vi "E5071C校准.vi"(4 "起始频率":dbl=947500000.0 format="%^.2e", 6 "测量点数":i32=401, 7 "终止频率":dbl=200000000.0 format="%^.2e", 9 "中频带宽":dbl=10000.0 format="%^.2e", 10 "Save State (F: Disable)":bool, 11 "VISA Refnum in":refnum<visa-resource-name>) -> ()   [LabVIEW 2011]
uses:
  Agilent ENA Series/Agilent ENA Series.lvlib
panel:
  # "kHz"
  # "MHz"
  # "MHz"
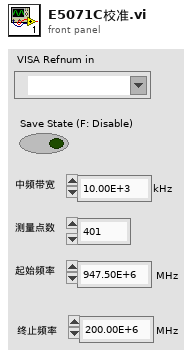
[diagram p1: front panel]
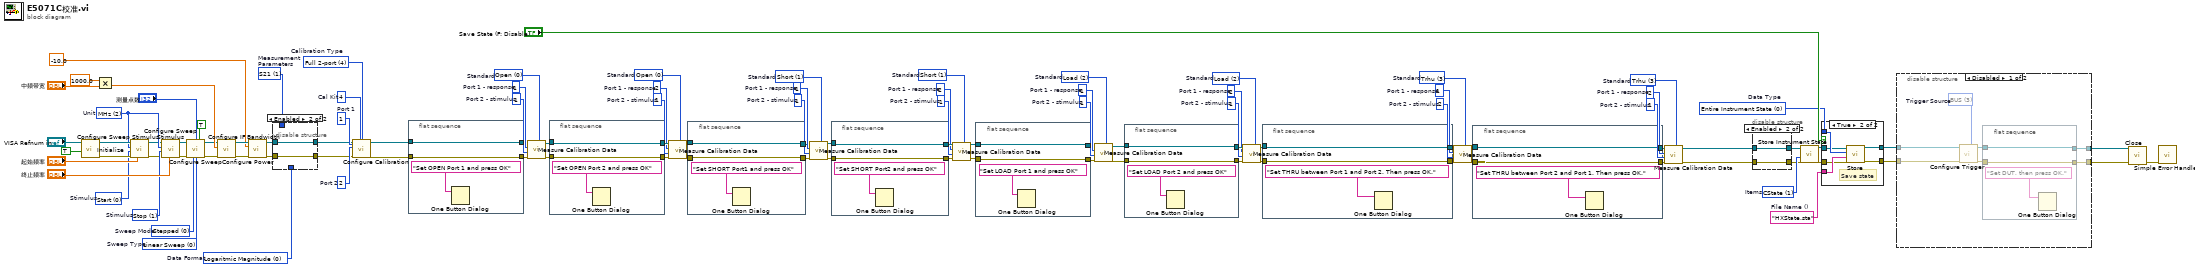
[diagram p0: block diagram]
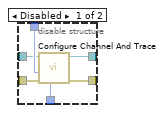
[diagram p2: hidden frame]
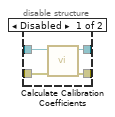
[diagram p4: hidden frame]
diagram:
  w89 = "HXState.sta"  # File Name ()
  w88 = u16 0 items=["Entire Instrument State", "Formatted Data Array", "Image On The LCD Display", "Segment Sweep Table", "Limit Table", "Power Sensor A", "Power Sensor B", "VBA Project", "Loss Compensation Table 1", "Loss Compensation Table 2", "Loss Compensation Table 3", "Loss Compensation Table 4"]  # Data Type
  w102 = u16 1 items=["State", "CState", "Dstate", "CDState"]  # Items
  w81 = u16 3 items=["Open", "Short", "Load", "Trhu", "Isolation"]  # Standard
  w79 = 1  # Port 2 - stimulus
  w80 = 2  # Port 1 - response
  w72 = u16 3 items=["Open", "Short", "Load", "Trhu", "Isolation"]  # Standard
  w76 = 2  # Port 2 - stimulus
  w75 = 1  # Port 1 - response
  w69 = u16 2 items=["Open", "Short", "Load", "Trhu", "Isolation"]  # Standard
  w65 = 1  # Port 2 - stimulus
  w66 = 2  # Port 1 - response
  w58 = u16 2 items=["Open", "Short", "Load", "Trhu", "Isolation"]  # Standard
  w62 = 1  # Port 2 - stimulus
  w61 = 1  # Port 1 - response
  w55 = u16 1 items=["Open", "Short", "Load", "Trhu", "Isolation"]  # Standard
  w51 = 1  # Port 2 - stimulus
  w52 = 2  # Port 1 - response
  w44 = u16 1 items=["Open", "Short", "Load", "Trhu", "Isolation"]  # Standard
  w48 = 1  # Port 2 - stimulus
  w47 = 1  # Port 1 - response
  w43 = u16 0 items=["Open", "Short", "Load", "Trhu", "Isolation"]  # Standard
  w42 = u16 0 items=["Open", "Short", "Load", "Trhu", "Isolation"]  # Standard
  w36 = 1  # Port 2 - stimulus
  w37 = 2  # Port 1 - response
  w35 = 1  # Port 2 - stimulus
  w34 = 1  # Port 1 - response
  w29 = 2  # Port 2
  w28 = 1  # Port 1
  w27 = u16 4 items=["Open", "Short", "Through", "1-port", "Full 2-port", "Full 3-port", "Full 4-port"]  # Calibration Type
  w26 = 4  # Cal Kit
  w23 = u16 0 items=["Logaritmic Magnitude", "Phase", "Group Delay", "Smith Chart  Linear (Lin/Phase)", "Smith Chart  Logaritmic (Log/Phase)", "Smith Chart  Complex (Real/Imag)", "Smith Chart  Impedance (R+jX)", "Smith Chart  Admittance (G+jB)", "Polar Format (Linear)", "Polar Format (Logaritmic)", "Polar Format (Re/Im)", "Linear Magnitude", "SWR", "Real", "Imaginary", "Epanded Phase", "Positive Phase"]  # Data Format
  w22 = u16 1 items=["S11", "S21", "S31", "S41", "S12", "S22", "S32", "S42", "S13", "S23", "S33", "S43", "S14", "S24", "S34", "S44", "A", "B", "C", "D", "R1", "R2", "R3", "R4"]  # Measurement Parameters
  w11 = u16 0 items=["Linear Sweep", "Logaritmic Sweep", "Segment Sweep", "Power Sweep"]  # Sweep Type
  w9 = u16 0 items=["Stepped", "Swept", "Fast Stepped Mode", "Fast Swept Mode"]  # Sweep Mode
  w6 = u16 1 items=["Start", "Stop", "Center", "Span"]  # Stimulus
  w8 = u16 2 items=["Hz", "kHz", "MHz", "GHz", "dBm", "s"]  # Unit
  w2 = u16 0 items=["Start", "Stop", "Center", "Span"]  # Stimulus
  n1 = call "Initialize.vi"("Reset? (T: Yes)"=TRUE, "VISA resource name"="VISA Refnum in") -> ("error out"=w87:errorcluster, "VISA resource name out"=w86:refnum<visa-resource-name>)  [unwired: 8 in]
  n2 = Multiply(x=1000.0, y="中频带宽") -> (x*y=w105:dbl)
  n3 = call "Configure Sweep Stimulus.vi"("Parameter (0.0)"="起始频率", "error in (no error)"=w87, "Stimulus (0: Start)"=w2, "Unit (0: Hz)"=w8, "VISA resource name"=w86) -> ("error out"=w4:errorcluster, "VISA resource name out"=w5:refnum<visa-resource-name>)  [unwired: 5 in]
  n4 = call "Configure Sweep Stimulus.vi"("Parameter (0.0)"="终止频率", "error in (no error)"=w4, "Stimulus (0: Start)"=w6, "Unit (0: Hz)"=w8, "VISA resource name"=w5) -> ("error out"=w12:errorcluster, "VISA resource name out"=w13:refnum<visa-resource-name>)  [unwired: 5 in]
  n5 = call "Configure Sweep.vi"("VISA resource name"=w13, "Number of Measurement Points (201)"="测量点数", "Auto Sweep Time (F: Off)"=TRUE, "error in (no error)"=w12, "Sweep Mode (0: Stepped)"=w9, "Sweep Type (0: Linear Sweep)"=w11) -> ("VISA resource name out"=w15:refnum<visa-resource-name>, "error out"=w16:errorcluster)  [unwired: 8 in]
  n6 = call "Configure IF Bandwidth.vi"("error in (no error)"=w16, "IF Bandwidth (100000.0)"=w105, "VISA resource name"=w15) -> ("error out"=w18:errorcluster, "VISA resource name out"=w19:refnum<visa-resource-name>)  [unwired: 7 in]
  n7 = call "Configure Power.vi"("VISA resource name"=w19, "Power Level (0.0)"=-10.0 ("Power (dBm)"), "error in (no error)"=w18) -> ("VISA resource name out"=w20:refnum<visa-resource-name>, "error out"=w21:errorcluster)  [unwired: 11 in]
  n8 = disable-structure shown="Enabled" {
    disable-tunnel: [w112 w113] -> w25
    disable-tunnel: [w111 w114] -> w24
    disable-tunnel: w23 -> [w110 _]
    disable-tunnel: w22 -> [w109 _]
    disable-tunnel: w21 -> [w108 w113]
    disable-tunnel: w20 -> [w107 w114]
    frame Disabled {
      n9 = call "Configure Channel And Trace.vi"("Data Format (0: Logarithmic Magnitude)"=w110, "error in (no error)"=w108, "Measurement Parameters (0: S11)"=w109, "VISA resource name"=w107) -> ("error out"=w112:errorcluster, "VISA resource name out"=w111:refnum<visa-resource-name>)  [unwired: 6 in]
    }
    frame Enabled {
    }
  }
  n10 = call "Configure Calibration.vi"("VISA resource name"=w24, "Port 1 (1)"=w28, "Port 2 (1)"=w29, "error in (no error)"=w25, "Cal Kit (1)"=w26, "Calibration Type (6: Full 4-port)"=w27) -> ("VISA resource name out"=w30:refnum<visa-resource-name>, "error out"=w31:errorcluster)  [unwired: 12 in]
  n11 = flat-sequence {
    tunnel: w30 -> [w116]
    tunnel: w31 -> [w115]
    tunnel: [w115] -> w33
    tunnel: [w116] -> w32
    frame #0 {
      n12 = One Button Dialog(message="Set OPEN Port 1 and press OK") -> ()  [unwired: 1 in, 1 out]
    }
  }
  n13 = call "Measure Calibration Data.vi"("Standard (0: Open)"=w42, "error in (no error)"=w33, "Port 2 - stimulus (2)"=w35, "Port 1 - response (1)"=w34, "VISA resource name"=w32) -> ("error out"=w41:errorcluster, "VISA resource name out"=w40:refnum<visa-resource-name>)  [unwired: 5 in]
  n14 = flat-sequence {
    tunnel: w40 -> [w119]
    tunnel: w41 -> [w118]
    tunnel: [w118] -> w38
    tunnel: [w119] -> w39
    frame #0 {
      n15 = One Button Dialog(message="Set OPEN Port 2 and press OK") -> ()  [unwired: 1 in, 1 out]
    }
  }
  n16 = call "Measure Calibration Data.vi"("Standard (0: Open)"=w43, "error in (no error)"=w38, "Port 2 - stimulus (2)"=w36, "Port 1 - response (1)"=w37, "VISA resource name"=w39) -> ("error out"=w50:errorcluster, "VISA resource name out"=w49:refnum<visa-resource-name>)  [unwired: 5 in]
  n17 = flat-sequence {
    tunnel: w49 -> [w122]
    tunnel: w50 -> [w121]
    tunnel: [w121] -> w46
    tunnel: [w122] -> w45
    frame #0 {
      n18 = One Button Dialog(message="Set SHORT Port1 and press OK") -> ()  [unwired: 1 in, 1 out]
    }
  }
  n19 = call "Measure Calibration Data.vi"("Standard (0: Open)"=w44, "error in (no error)"=w46, "Port 2 - stimulus (2)"=w48, "Port 1 - response (1)"=w47, "VISA resource name"=w45) -> ("error out"=w57:errorcluster, "VISA resource name out"=w56:refnum<visa-resource-name>)  [unwired: 5 in]
  n20 = flat-sequence {
    tunnel: w56 -> [w125]
    tunnel: w57 -> [w124]
    tunnel: [w124] -> w53
    tunnel: [w125] -> w54
    frame #0 {
      n21 = One Button Dialog(message="Set SHORT Port2 and press OK") -> ()  [unwired: 1 in, 1 out]
    }
  }
  n22 = call "Measure Calibration Data.vi"("Standard (0: Open)"=w55, "error in (no error)"=w53, "Port 2 - stimulus (2)"=w51, "Port 1 - response (1)"=w52, "VISA resource name"=w54) -> ("error out"=w64:errorcluster, "VISA resource name out"=w63:refnum<visa-resource-name>)  [unwired: 5 in]
  n23 = flat-sequence {
    tunnel: w63 -> [w128]
    tunnel: w64 -> [w127]
    tunnel: [w127] -> w60
    tunnel: [w128] -> w59
    frame #0 {
      n24 = One Button Dialog(message="Set LOAD Port 1 and press OK") -> ()  [unwired: 1 in, 1 out]
    }
  }
  n25 = call "Measure Calibration Data.vi"("Standard (0: Open)"=w58, "error in (no error)"=w60, "Port 2 - stimulus (2)"=w62, "Port 1 - response (1)"=w61, "VISA resource name"=w59) -> ("error out"=w71:errorcluster, "VISA resource name out"=w70:refnum<visa-resource-name>)  [unwired: 5 in]
  n26 = flat-sequence {
    tunnel: w70 -> [w131]
    tunnel: w71 -> [w130]
    tunnel: [w130] -> w67
    tunnel: [w131] -> w68
    frame #0 {
      n27 = One Button Dialog(message="Set LOAD Port 2 and press OK") -> ()  [unwired: 1 in, 1 out]
    }
  }
  n28 = call "Measure Calibration Data.vi"("Standard (0: Open)"=w69, "error in (no error)"=w67, "Port 2 - stimulus (2)"=w65, "Port 1 - response (1)"=w66, "VISA resource name"=w68) -> ("error out"=w78:errorcluster, "VISA resource name out"=w77:refnum<visa-resource-name>)  [unwired: 5 in]
  n29 = flat-sequence {
    tunnel: w77 -> [w134]
    tunnel: w78 -> [w133]
    tunnel: [w133] -> w74
    tunnel: [w134] -> w73
    frame #0 {
      n30 = One Button Dialog(message="Set THRU between Port 1 and Port 2. Then press OK.") -> ()  [unwired: 1 in, 1 out]
    }
  }
  n31 = call "Measure Calibration Data.vi"("Standard (0: Open)"=w72, "error in (no error)"=w74, "Port 2 - stimulus (2)"=w76, "Port 1 - response (1)"=w75, "VISA resource name"=w73) -> ("error out"=w83:errorcluster, "VISA resource name out"=w82:refnum<visa-resource-name>)  [unwired: 5 in]
  n32 = flat-sequence {
    tunnel: w82 -> [w137]
    tunnel: w83 -> [w136]
    tunnel: [w136] -> w94
    tunnel: [w137] -> w93
    frame #0 {
      n33 = One Button Dialog(message="Set THRU between Port 2 and Port 1. Then press OK.") -> ()  [unwired: 1 in, 1 out]
    }
  }
  n34 = call "Measure Calibration Data.vi"("Standard (0: Open)"=w81, "error in (no error)"=w94, "Port 2 - stimulus (2)"=w79, "Port 1 - response (1)"=w80, "VISA resource name"=w93) -> ("error out"=w97:errorcluster, "VISA resource name out"=w96:refnum<visa-resource-name>)  [unwired: 5 in]
  n35 = disable-structure shown="Enabled" {
    disable-tunnel: w96 -> [w142 w144]
    disable-tunnel: w97 -> [w141 w143]
    disable-tunnel: [w140 w143] -> w98
    disable-tunnel: [w139 w144] -> w99
    frame Disabled {
      n36 = call "Calculate Calibration Coefficients.vi"("error in (no error)"=w141, "VISA resource name"=w142) -> ("error out"=w140:errorcluster, "VISA resource name out"=w139:refnum<visa-resource-name>)  [unwired: 8 in]
    }
    frame Enabled {
    }
  }
  n37 = call "Store Instrument State.vi"("error in (no error)"=w98, "Items (1: CState)"=w102, "VISA resource name"=w99) -> ("error out"=w101:errorcluster, "VISA resource name out"=w100:refnum<visa-resource-name>)  [unwired: 7 in]
  n38 = case shown="True" "Save State (F: Disable)" {
    tunnel: w88 -> [_ w152]
    tunnel: w89 -> [_ w151]
    tunnel: w100 -> [w146 w150]
    tunnel: [w146 w149] -> w90
    tunnel: w101 -> [w145 w148]
    tunnel: [w145 w147] -> w91
    frame False {
      # "Don't save"
    }
    frame True {
      # "Save state"
      n39 = call "Store.vi"("error in (no error)"=w148, "File Name ()"=w151, "Data Type (0: Entire Instrument State)"=w152, "VISA resource name"=w150) -> ("error out"=w147:errorcluster, "VISA resource name out"=w149:refnum<visa-resource-name>)  [unwired: 6 in]
    }
  }
  n40 = disable-structure shown="Disabled" {
    disable-tunnel: [w159 w163] -> w104
    disable-tunnel: [w158 w164] -> w103
    disable-tunnel: w91 -> [w157 w163]
    disable-tunnel: w90 -> [w156 w164]
    frame Disabled {
      w153 = u16 3 items=["Internal", "External", "Manual", "BUS"]  # Trigger Source
      n41 = call "Configure Trigger.vi"("Trigger Source (0: Internal)"=w153, "error in (no error)"=w157, "VISA resource name"=w156) -> ("error out"=w155:errorcluster, "VISA resource name out"=w154:refnum<visa-resource-name>)  [unwired: 7 in]
      n42 = flat-sequence {
        tunnel: w154 -> [w160]
        tunnel: w155 -> [w161]
        tunnel: [w161] -> w159
        tunnel: [w160] -> w158
        frame #0 {
          n43 = One Button Dialog(message="Set DUT, then press OK.") -> ()  [unwired: 1 in, 1 out]
        }
      }
    }
    frame Enabled {
    }
  }
  n44 = call "Close.vi"("error in (no error)"=w104, "VISA resource name"=w103) -> ("error out"=w84:errorcluster)  [unwired: 9 in]
  n45 = call <vilib>:"Simple Error Handler.vi"("error in (no error)"=w84) -> ()  [unwired: 4 in, 5 out]
